vi "testReadSinglePoint.vi"(8 "error in (no error)":errorcluster, 11 "TestCase in":refnum<class "Pointer Tests.lvclass">) -> (0 "error out":errorcluster, 3 "TestCase out":refnum<class "Pointer Tests.lvclass">)   [LabVIEW 2017]
uses:
  Pointer Tests.lvclass
  <vilib>/addons/_JKI Toolkits/VI Tester/TestCase.llb/TestCase.lvclass
  C:/Program Files (x86)/National Instruments/LabVIEW 2017/vi.lib/addons/_JKI Toolkits/VI Tester/TestCase.llb/TestCase.lvclass
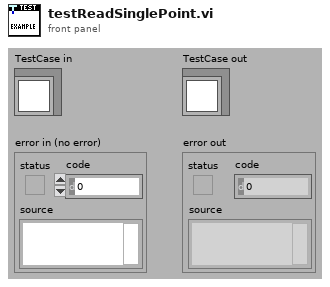
[diagram p1: front panel]
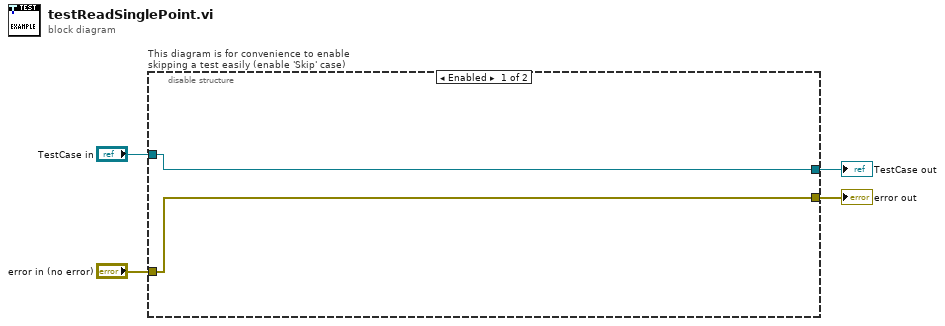
[diagram p0: block diagram]
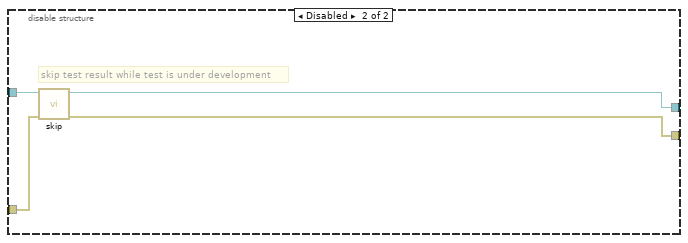
[diagram p2: hidden frame]
diagram:
  n1 = disable-structure "This diagram is for convenience to enable skipping a test easily (enable 'Skip' case)" shown="Enabled" {
    disable-tunnel: "TestCase in" -> [w5 w10]
    disable-tunnel: [w5 w8] -> w1
    disable-tunnel: [w6 w9] -> w3
    disable-tunnel: "error in (no error)" -> [w6 w7]
    frame Enabled {
    }
    frame Disabled {
      # "skip test result while test is under development"
      n2 = call <vilib>:"skip.vi"("error in (no error)"=w7, "TestCase in"=w10) -> ("error out"=w9:errorcluster, "TestCase out"=w8:refnum<class "Pointer Tests.lvclass">)  [unwired: 8 in]
    }
  }
  "error out" <- w3
  "TestCase out" <- w1
